vi "REPORT.Max Min P N.vi"(9 "Vasic":i32, 10 "Test":T1={"Config HW"={"VISA Rigol DP832"="Rigol_DP832", "Config Rigol DP832"=[{"Channel"=0, "V Limit"=5.5, "I Limit"=0.5, "V Out"=5.0}, {"Channel"=1, "V Limit"=5.5, "I Limit"=0.8, "V Out"=5.0}, {"Channel"=2, "V Limit"=5.5, "I Limit"=0.2, "V Out"=0.0}], "CTA Test#"="CTA013 A", "FT_Handle"=0, "Espera acceso FT"=10, "VISA Tek MDO3104"="Rigol_DP832", "VISA Key 81160A"="Rigol_DP832"}, "Config Test"=[{"Vasic"=2.8, "Global Reset"=FALSE, "Test Register?"=FALSE, "Test ADC?"=FALSE, "Test ADC"={"Repeats ADC"=100, "Max Desviation"=0.1}, "Limits ADC"={"Low"=[1.9, 1.3, 0.65, 0.0, 1.6, 1.4, 1.4, 0.9, 2.1, 0.85, 1.9], "High"=[2.1, 1.5, 0.85, 0.1, 1.4, 1.2, 1.2, 0.7, 1.9, 0.65, 1.7]}, "Test Max PN Min NP?"=FALSE, "Limits Max PN Min NP"={"Max P Upper"=2.177000045776367, "Min P Upper"=1.474, "Max N Upper"=1.475, "Min N Upper"=0.818, "Max P Lower"=1.888, "Min P Lower "=1.321, "Max N Lower"=1.322, "Min N Lower"=0.73}, "Test Rate Scan?"=FALSE, "Vin Rate Scan"=[], "Limits Rate Scan"={"High"=[0.15, 0.242, 0.331, 0.425, 0.512, 0.6, 0.688, 0.774, 0.847, 0.91], "Low"=[0.021, 0.11, 0.189, 0.27, 0.347, 0.421, 0.487, 0.551, 0.601, 0.635]}, "Test Rate Scan Adders?"=FALSE, "Vin Rate Adders"=[], "Limits Rate Scan adders"={"High"=[], "Low"=[]}, "Test offset analog?"=FALSE, "Lim Offset Analog"={"Max Analog"=0.05, "Min Analog"=-0.05}, "Test offset digital?"=FALSE, "Lim offset Dig"={"Max Dig"=0.05}, "Vasic real f.a."=2.8, "IBIAS"=FALSE, "VALUE IBIAS"=63}, {"Vasic"=2.8, "Global Reset"=FALSE, "Test Register?"=FALSE, "Test ADC?"=FALSE, "Test ADC"={"Repeats ADC"=100, "Max Desviation"=0.1}, "Limits ADC"={"Low"=[1.9, 1.3, 0.65, 0.0, 1.6, 1.4, 1.4, 0.9, 2.1, 0.85, 1.9], "High"=[2.1, 1.5, 0.85, 0.1, 1.4, 1.2, 1.2, 0.7, 1.9, 0.65, 1.7]}, "Test Max PN Min NP?"=FALSE, "Limits Max PN Min NP"={"Max P Upper"=2.177000045776367, "Min P Upper"=1.474, "Max N Upper"=1.475, "Min N Upper"=0.818, "Max P Lower"=1.888, "Min P Lower "=1.321, "Max N Lower"=1.322, "Min N Lower"=0.73}, "Test Rate Scan?"=FALSE, "Vin Rate Scan"=[], "Limits Rate Scan"={"High"=[0.15, 0.242, 0.331, 0.425, 0.512, 0.6, 0.688, 0.774, 0.847, 0.91], "Low"=[0.021, 0.11, 0.189, 0.27, 0.347, 0.421, 0.487, 0.551, 0.601, 0.635]}, "Test Rate Scan Adders?"=FALSE, "Vin Rate Adders"=[], "Limits Rate Scan adders"={"High"=[], "Low"=[]}, "Test offset analog?"=FALSE, "Lim Offset Analog"={"Max Analog"=0.05, "Min Analog"=-0.05}, "Test offset digital?"=FALSE, "Lim offset Dig"={"Max Dig"=0.05}, "Vasic real f.a."=2.8, "IBIAS"=FALSE, "VALUE IBIAS"=63}, {"Vasic"=2.8, "Global Reset"=FALSE, "Test Register?"=FALSE, "Test ADC?"=FALSE, "Test ADC"={"Repeats ADC"=100, "Max Desviation"=0.1}, "Limits ADC"={"Low"=[1.9, 1.3, 0.65, 0.0, 1.6, 1.4, 1.4, 0.9, 2.1, 0.85, 1.9], "High"=[2.1, 1.5, 0.85, 0.1, 1.4, 1.2, 1.2, 0.7, 1.9, 0.65, 1.7]}, "Test Max PN Min NP?"=FALSE, "Limits Max PN Min NP"={"Max P Upper"=2.177000045776367, "Min P Upper"=1.474, "Max N Upper"=1.475, "Min N Upper"=0.818, "Max P Lower"=1.888, "Min P Lower "=1.321, "Max N Lower"=1.322, "Min N Lower"=0.73}, "Test Rate Scan?"=FALSE, "Vin Rate Scan"=[], "Limits Rate Scan"={"High"=[0.15, 0.242, 0.331, 0.425, 0.512, 0.6, 0.688, 0.774, 0.847, 0.91], "Low"=[0.021, 0.11, 0.189, 0.27, 0.347, 0.421, 0.487, 0.551, 0.601, 0.635]}, "Test Rate Scan Adders?"=FALSE, "Vin Rate Adders"=[], "Limits Rate Scan adders"={"High"=[], "Low"=[]}, "Test offset analog?"=FALSE, "Lim Offset Analog"={"Max Analog"=0.05, "Min Analog"=-0.05}, "Test offset digital?"=FALSE, "Lim offset Dig"={"Max Dig"=0.05}, "Vasic real f.a."=2.8, "IBIAS"=FALSE, "VALUE IBIAS"=63}, {"Vasic"=2.8, "Global Reset"=FALSE, "Test Register?"=FALSE, "Test ADC?"=FALSE, "Test ADC"={"Repeats ADC"=100, "Max Desviation"=0.1}, "Limits ADC"={"Low"=[1.9, 1.3, 0.65, 0.0, 1.6, 1.4, 1.4, 0.9, 2.1, 0.85, 1.9], "High"=[2.1, 1.5, 0.85, 0.1, 1.4, 1.2, 1.2, 0.7, 1.9, 0.65, 1.7]}, "Test Max PN Min NP?"=FALSE, "Limits Max PN Min NP"={"Max P Upper"=2.177000045776367, "Min P Upper"=1.474, "Max N Upper"=1.475, "Min N Upper"=0.818, "Max P Lower"=1.888, "Min P Lower "=1.321, "Max N Lower"=1.322, "Min N Lower"=0.73}, "Test Rate Scan?"=FALSE, "Vin Rate Scan"=[], "Limits Rate Scan"={"High"=[0.15, 0.242, 0.331, 0.425, 0.512, 0.6, 0.688, 0.774, 0.847, 0.91], "Low"=[0.021, 0.11, 0.189, 0.27, 0.347, 0.421, 0.487, 0.551, 0.601, 0.635]}, "Test Rate Scan Adders?"=FALSE, "Vin Rate Adders"=[], "Limits Rate Scan adders"={"High"=[], "Low"=[]}, "Test offset analog?"=FALSE, "Lim Offset Analog"={"Max Analog"=0.05, "Min Analog"=-0.05}, "Test offset digital?"=FALSE, "Lim offset Dig"={"Max Dig"=0.05}, "Vasic real f.a."=2.8, "IBIAS"=FALSE, "VALUE IBIAS"=63}], "Result"=[], "Execucion Test"={"Vasic Actual"=0}, "Config VGA"={"Theoretical Voltage"=[], "Real Voltage"=[], "Pulse Width"=57344, "Frecuency Pulse"=1000000.0, "VGA Gain"=[]}, "Test Info"={"Asic"="", "Operator"="", "Place"="", "Time start"=timestamp(0 s since 1904-01-01), "Time stop"=timestamp(0 s since 1904-01-01)}, "Info machine"={"SO"="", "SO Name"="", "SO Ver"="", "SO Build"="", "CPU"="", "APP"="", "APP YEAR"="", "APP ver"="", "APP User"="", "APP Serail"="", "MAC"=[], "PC NAME"=[], "PC IP"=[], "BIOS MANU"="", "BIOS NAME"="", "BIOS SERIAL"="", "BOARD MANU"="", "BOARD NAME"="", "BOARD SERIAL"="", "Driver Version"="", "Library Version"="", "FPGA Ver"=0, "ID CTA board"=0, "LAST BOOT"="", "LABVIEW Ver"=0}, "Partial Report"="", "CONFIG GEN"=[]} {"CONFIG GEN"."Vasic Theorical" min=1.0 max=1000000.0 step=1.0 format="%#_6pV"; "CONFIG GEN"."Frequency" min=0.001 max=333000000.0 step=1000.0 format="%#_6pHz"; "CONFIG GEN"."Leading Edge Time" min=1e-09 max=1.0 step=1e-10 format="%#_6ps"; "CONFIG GEN"."Trailing Edge Time" min=1e-09 max=1.0 step=1e-10 format="%#_6ps"; "CONFIG GEN"."Delay" min=0.0 max=1.0 step=1e-12 format="%#_6ps"; "CONFIG GEN"."Trigger Level Sync" items=["ECL", "TTL"]; "CONFIG GEN"."Trigger Sync Out" items=["AB"=3, "B"=2, "A"=1, "None"=0]; "CONFIG GEN"."Load" min=1.0 max=1000000.0 step=1.0 format="%#_6p"; "CONFIG GEN"."DC Offset" min=-10.0 max=10.0 step=0.1 format="%#_6pV"; "CONFIG GEN"."Amplitude" min=0.05 max=5.0 step=0.001 format="%#_6pV"; "CONFIG GEN"."Width Time" min=1.5e-09 max=1.0 step=1e-10 format="%#_6ps"; "CONFIG GEN"."Channel" items=["Channel1"=1, "Channel2"=2]; "Config VGA"."Theoretical Voltage" format="%1.4f"; "Config VGA"."VGA Gain" format="%02x"; "Config VGA"."Frecuency Pulse" format="%0_2p"; "Config VGA"."Pulse Width" format="%04x"; "Config VGA"."Real Voltage" format="%1.5f"; "Config Test"."VALUE IBIAS" max=63 step=1; "Config Test"."Vasic real f.a." min=2.8 max=3.8 step=0.01 format="%.2g"; "Config Test"."Limits Rate Scan adders"."Low" format="%1.3f"; "Config Test"."Limits Rate Scan adders"."High" format="%1.3f"; "Config Test"."Limits ADC"."High" format="%1.4f"; "Config Test"."Limits ADC"."Low" format="%1.3f"; "Config Test"."Lim offset Dig"."Max Dig" format="%.3g"; "Config Test"."Lim Offset Analog"."Min Analog" format="%.3g"; "Config Test"."Lim Offset Analog"."Max Analog" format="%.3g"; "Config Test"."Limits Rate Scan"."Low" format="%1.4f"; "Config Test"."Limits Rate Scan"."High" format="%1.3f"; "Config Test"."Limits Max PN Min NP"."Min P Upper" format="%.3g"; "Config Test"."Limits Max PN Min NP"."Min P Lower" format="%.3g"; "Config Test"."Limits Max PN Min NP"."Max N Lower" format="%.3g"; "Config Test"."Limits Max PN Min NP"."Max N Upper" format="%.3g"; "Config Test"."Limits Max PN Min NP"."Min N Lower" format="%.3g"; "Config Test"."Limits Max PN Min NP"."Min N Upper" format="%.3g"; "Config Test"."Limits Max PN Min NP"."Max P Upper" format="%.3g"; "Config Test"."Limits Max PN Min NP"."Max P Lower" format="%.3g"; "Config Test"."Vasic" min=2.8 max=3.8 step=0.01 format="%.2g"; "Config HW"."Config Rigol DP832"."Channel" items=["+30V Channel 1", "+30V Channel 2", "+5V Channel 3"]; "Config HW"."Config Rigol DP832"."V Limit" format="%.1g"; "Config HW"."Config Rigol DP832"."I Limit" format="%.1g"; "Config HW"."Config Rigol DP832"."V Out" format="%.1g"; "Result"."Test Registros"."Read W/R" format="%04x"; "Result"."Test Registros"."Pattern W/R" format="%04x"; "Result"."Test Registros"."Read Default" format="%04x"; "Result"."Test Registros"."Pattern Default" format="%04x"}, 11 "Text in":string) -> (3 "Text Out":string)   [LabVIEW 2019]
uses:
  Test.ctl
  TEST.TEST CONFIG HW.ctl
  Rigol DP832/DP832_Control Channels.ctl
  TEST.TEST CONFIG TEST MATRIZ.ctl
  TEST.TEST CONFIG TEST.ctl
  TEST.TEST RESULT.ctl
  test_result fvasic.ctl
  TEST.TEST EXECUTION TEST.ctl
  TEST.TEST CONFIG VGA.ctl
  TEST.TEST TEST INFO.ctl
  TEST.TEST INFO PC.ctl
  GenPulse_configurar.ctl
panel:
  # "Modo 2\nModo 3\nModo 4\nModo 2\nModo 3\nModo 4"
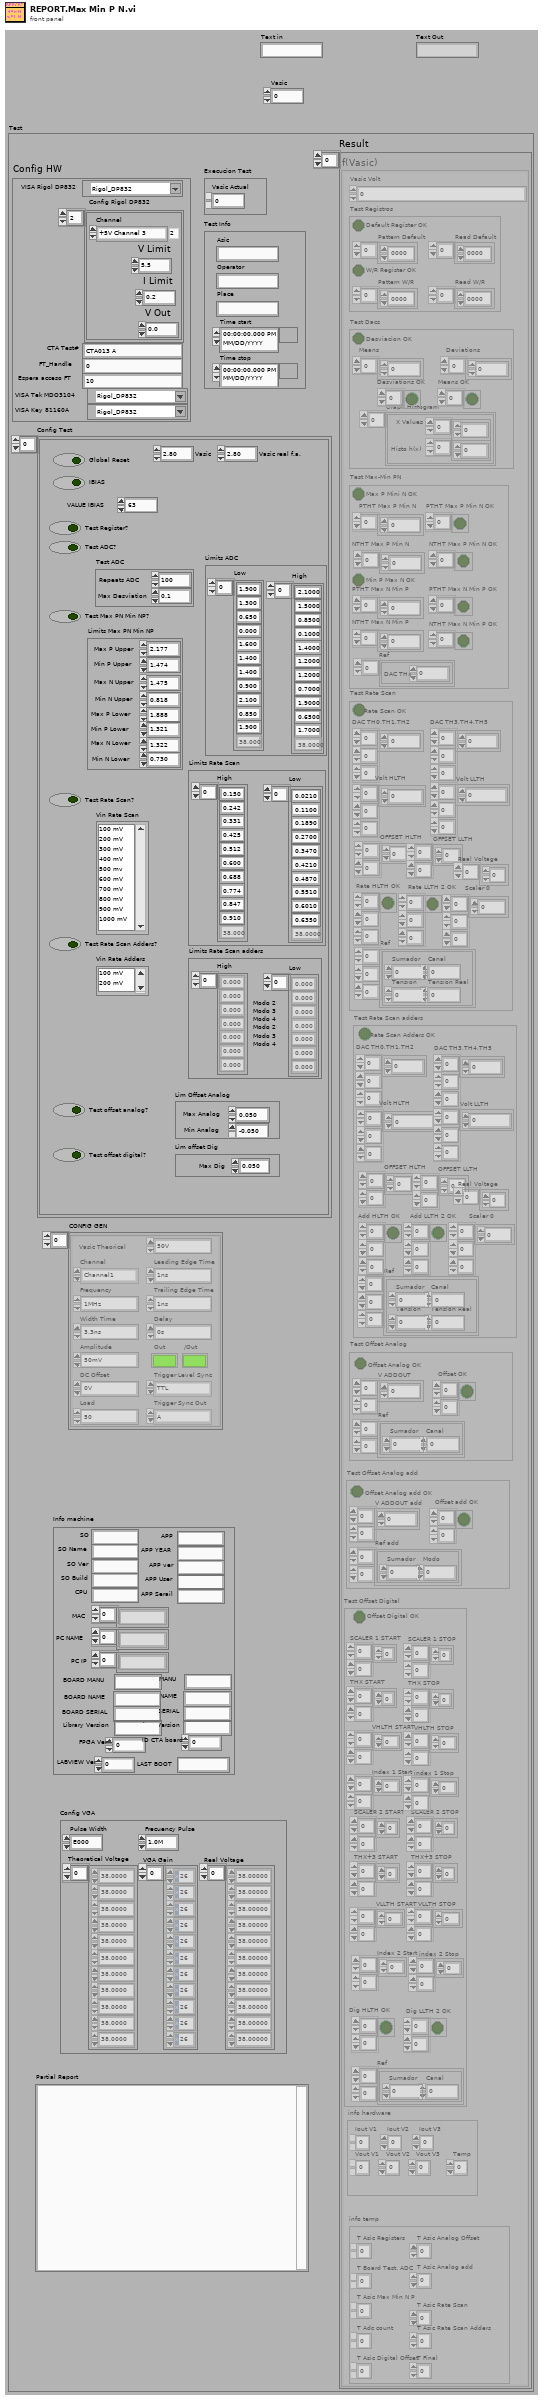
[diagram p1: front panel]
types:
  T1 = typedef "Test.ctl" = cluster{"Config HW":T2, "Config Test":T4, "Result":T6, "Execucion Test":T8, "Config VGA":T9, "Test Info":T10, "Info machine":T11, "Partial Report":string, "CONFIG GEN":T12[]}
  T2 = typedef "TEST.TEST CONFIG HW.ctl" = cluster{"VISA Rigol DP832":refnum<visa-resource-name>, "Config Rigol DP832":cluster{"Channel":T3, "V Limit":dbl, "I Limit":dbl, "V Out":dbl}[], "CTA Test#":string, "FT_Handle":u32, "Espera acceso FT":u32, "VISA Tek MDO3104":refnum<visa-resource-name>, "VISA Key 81160A":refnum<visa-resource-name>}
  T3 = typedef "DP832_Control Channels.ctl" = i32
  T4 = typedef "TEST.TEST CONFIG TEST MATRIZ.ctl" = T5[]
  T5 = typedef "TEST.TEST CONFIG TEST.ctl" = cluster{"Vasic":dbl, "Global Reset":bool, "Test Register?":bool, "Test ADC?":bool, "Test ADC":cluster{"Repeats ADC":i32, "Max Desviation":dbl}, "Limits ADC":cluster{"Low":dbl[], "High":dbl[]}, "Test Max PN Min NP?":bool, "Limits Max PN Min NP":cluster{"Max P Upper":dbl, "Min P Upper":dbl, "Max N Upper":dbl, "Min N Upper":dbl, "Max P Lower":dbl, "Min P Lower ":dbl, "Max N Lower":dbl, "Min N Lower":dbl}, "Test Rate Scan?":bool, "Vin Rate Scan":i32[], "Limits Rate Scan":cluster{"High":dbl[], "Low":dbl[]}, "Test Rate Scan Adders?":bool, "Vin Rate Adders":i32[], "Limits Rate Scan adders":cluster{"High":dbl[], "Low":dbl[]}, "Test offset analog?":bool, "Lim Offset Analog":cluster{"Max Analog":dbl, "Min Analog":dbl}, "Test offset digital?":bool, "Lim offset Dig":cluster{"Max Dig":dbl}, "Vasic real f.a.":dbl, "IBIAS":bool, "VALUE IBIAS":u8}
  T6 = typedef "TEST.TEST RESULT.ctl" = T7[]
  T7 = typedef "test_result fvasic.ctl" = cluster{"Vasic Volt":i32, "Test Registros":cluster{"Default Register OK":bool, "Pattern Default":u16[], "Read Default":u16[], "W/R Register OK":bool, "Pattern W/R":u16[], "Read W/R":u16[]}, "Test Dacs":cluster{"Desviacion OK":bool, "Means":dbl[], "Deviations":dbl[], "Desviations OK":bool[], "Means OK":bool[], "Graph Histogram":cluster{"X Values":dbl[], "Histo h(x)":i32[]}[]}, "Test Max-Min PN":cluster{"Max P Mini N OK":bool, "PTHT Max P Min N":dbl[], "PTHT Max P Min N OK":bool[], "NTHT Max P Min N":dbl[], "NTHT Max P Min N OK":bool[], "Min P Max N OK":bool, "PTHT Max N Min P":dbl[], "PTHT Max N Min P OK":bool[], "NTHT Max N Min P":dbl[], "NTHT Max N Min P OK":bool[], "Ref":cluster{"DAC THx":u8}[]}, "Test Rate Scan":cluster{"Rate Scan OK":bool, "DAC TH0,TH1,TH2":u16[][][], "Volt HLTH":dbl[][][], "Rate HLTH OK":bool[][][], "DAC TH3,TH4,TH5":u16[][][], "Volt LLTH":dbl[][][], "Rate LLTH 2 OK":bool[][][], "Scaler 0":u16[][][], "Ref":cluster{"Sumador":u8, "Canal":u8, "Tension":u8, "Tension Real":dbl}[][][], "OFFSET HLTH":dbl[][], "OFFSET LLTH":dbl[][], "Real Voltage":dbl[]}, "Test Rate Scan adders":cluster{"Rate Scan Adders OK":bool, "DAC TH0,TH1,TH2":u16[][][], "Volt HLTH":dbl[][][], "Add HLTH OK":bool[][][], "DAC TH3,TH4,TH5":u16[][][], "Volt LLTH":dbl[][][], "Add LLTH 2 OK":bool[][][], "Scaler 0":u16[][][], "Ref":cluster{"Sumador":u8, "Canal":u8, "Tension":u8, "Tension Real":dbl}[][][], "OFFSET HLTH":dbl[][], "OFFSET LLTH":dbl[][], "Real Voltage":dbl[]}, "Test Offset Analog":cluster{"Offset Analog OK":bool, "V ADDOUT":dbl[][], "Offset OK":bool[][], "Ref":cluster{"Sumador":u8, "Canal":u8}[][]}, "Test Offset Digital":cluster{"Offset Digital OK":bool, "SCALER 1 START":u16[][], "SCALER 1 STOP":u16[][], "THX START":u16[][], "THX STOP":u16[][], "VHLTH START":dbl[][], "VHLTH STOP":dbl[][], "Index 1 Start":i32[][], "index 1 Stop":i32[][], "SCALER 2 START":u16[][], "SCALER 2 STOP":u16[][], "THX+3 START":u16[][], "THX+3 STOP":u16[][], "VLLTH START":dbl[][], "VLLTH STOP":dbl[][], "Index 2 Start":i32[][], "index 2 Stop":i32[][], "Dig HLTH OK":bool[][], "Dig LLTH 2 OK":bool[][], "Ref":cluster{"Sumador":u8, "Canal":u8}[][]}, "info hardware":cluster{"Iout V1":dbl, "Iout V2":dbl, "Iout V3":dbl, "Vout V1":dbl, "Vout V2":dbl, "Vout V3":dbl, "Temp":dbl}, "Test Offset Analog add":cluster{"Offset Analog add OK":bool, "V ADDOUT add":dbl[][], "Offset add OK":bool[][], "Ref add":cluster{"Sumador":u8, "Modo":u8}[][]}, "info temp":cluster{"T Asic Registers":dbl, "T Board Test. ADC":dbl, "T Asic Max Min N P":dbl, "T Adc count":dbl, "T Asic Digital Offset":dbl, "T Asic Analog Offset":dbl, "T Asic Analog add":dbl, "T Asic Rate Scan":dbl, "T Asic Rate Scan Adders":dbl, "T Final":dbl}}
  T8 = typedef "TEST.TEST EXECUTION TEST.ctl" = cluster{"Vasic Actual":i32}
  T9 = typedef "TEST.TEST CONFIG VGA.ctl" = cluster{"Theoretical Voltage":dbl[], "Real Voltage":dbl[], "Pulse Width":u16, "Frecuency Pulse":dbl, "VGA Gain":u8[]}
  T10 = typedef "TEST.TEST TEST INFO.ctl" = cluster{"Asic":string, "Operator":string, "Place":string, "Time start":timestamp, "Time stop":timestamp}
  T11 = typedef "TEST.TEST INFO PC.ctl" = cluster{"SO":string, "SO Name":string, "SO Ver":string, "SO Build":string, "CPU":string, "APP":string, "APP YEAR":string, "APP ver":string, "APP User":string, "APP Serail":string, "MAC":string[], "PC NAME":string[], "PC IP":string[], "BIOS MANU":string, "BIOS NAME":string, "BIOS SERIAL":string, "BOARD MANU":string, "BOARD NAME":string, "BOARD SERIAL":string, "Driver Version":string, "Library Version":string, "FPGA Ver":u8, "ID CTA board":u64, "LAST BOOT":string, "LABVIEW Ver":u32}
  T12 = typedef "GenPulse_configurar.ctl" = cluster{"Channel":u16, "Frequency":dbl, "Width Time":dbl, "Amplitude":dbl, "DC Offset":dbl, "Load":dbl, "Leading Edge Time":dbl, "Trailing Edge Time":dbl, "Delay":dbl, "Out":bool, "/Out":bool, "Trigger Level Sync":u16, "Trigger Sync Out":u16, "Vasic Theorical":dbl}
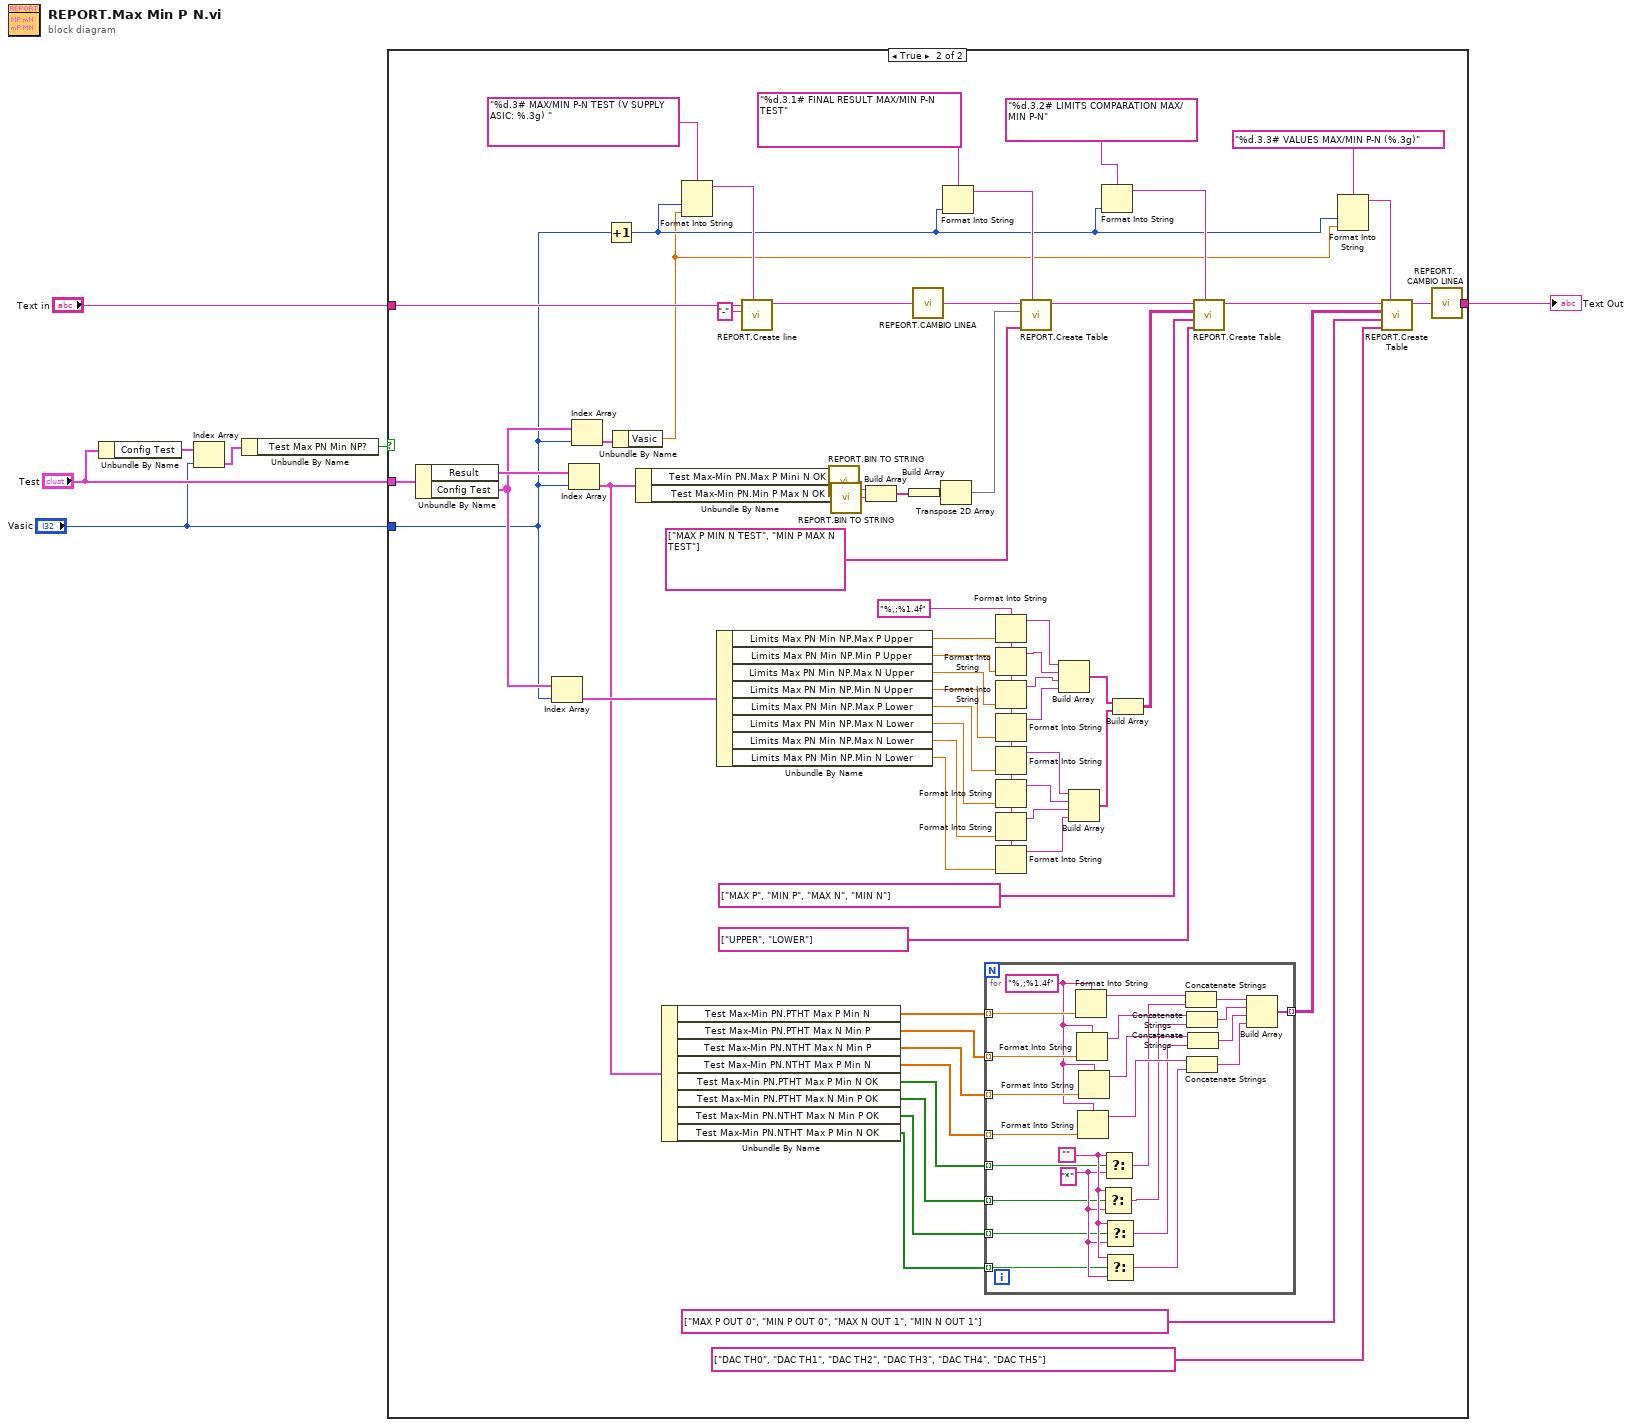
[diagram p0: block diagram]
diagram:
  n1 = Unbundle By Name("Test") -> ("Config Test"=w5:T4)
  n2 = Index Array(array=w5, index="Vasic") -> (element=w4:T5)
  n3 = Unbundle By Name(w4) -> ("Test Max PN Min NP?"=w1:bool)
  n4 = case shown="True" w1 {
    tunnel: "Text in" -> [w8 w68]
    tunnel: [w8 w24] -> w6
    tunnel: "Test" -> [_ w12]
    tunnel: "Vasic" -> [_ w11]
    frame False {
    }
    frame True {
      w43 = "%,;%1.4f" ("format string")
      n5 = Unbundle By Name(w12) -> ("Result"=w67:T6, "Config Test"=w19:T4)
      n6 = Index Array(array=w19, index=w11) -> (element=w64:T5)
      n7 = Index Array(array=w67, index=w11) -> (element=w39:T7)
      n8 = Index Array(array=w19, index=w11) -> (element=w18:T5)
      n9 = Increment(x=w11) -> (x+1=w13:i32)
      n10 = Unbundle By Name(w18) -> ("Vasic"=w10:dbl)
      n11 = Unbundle By Name(w39) -> ("Test Max-Min PN.Max P Mini N OK"=w72:bool, "Test Max-Min PN.Min P Max N OK"=w73:bool)
      n12 = Unbundle By Name(w39) -> ("Test Max-Min PN.PTHT Max P Min N"=w38:dbl[], "Test Max-Min PN.PTHT Max N Min P"=w37:dbl[], "Test Max-Min PN.NTHT Max N Min P"=w36:dbl[], "Test Max-Min PN.NTHT Max P Min N"=w35:dbl[], "Test Max-Min PN.PTHT Max P Min N OK"=w31:bool[], "Test Max-Min PN.PTHT Max N Min P OK"=w30:bool[], "Test Max-Min PN.NTHT Max N Min P OK"=w29:bool[], "Test Max-Min PN.NTHT Max P Min N OK"=w28:bool[])
      n13 = Format Into String(format string="%d.3# MAX/MIN P-N TEST (V SUPPLY ASIC: %.3g) " ("Secction"), w13, w10) -> (resulting string=w17:string)  [unwired: 2 in, 1 out]
      n14 = Unbundle By Name(w64) -> ("Limits Max PN Min NP.Max P Upper"=w63:dbl, "Limits Max PN Min NP.Min P Upper"=w62:dbl, "Limits Max PN Min NP.Max N Upper"=w61:dbl, "Limits Max PN Min NP.Min N Upper"=w60:dbl, "Limits Max PN Min NP.Max P Lower"=w59:dbl, "Limits Max PN Min NP.Max N Lower"=w58:dbl, "Limits Max PN Min NP.Max N Lower"=w57:dbl, "Limits Max PN Min NP.Min N Lower"=w56:dbl)
      n15 = call "REPORT.Create line.vi"("Secction"=w17, "Char"="-", "Text In"=w68) -> ("Text Out"=w55:string)  [unwired: 8 in]
      n16 = call "REPORT.BIN TO STRING.vi"("Resultado test"=w72) -> ("OK, Fault"=w71:string)  [unwired: 14 in]
      n17 = call "REPORT.BIN TO STRING.vi"("Resultado test"=w73) -> ("OK, Fault"=w70:string)  [unwired: 14 in]
      n18 = Build Array(w71, w70) -> (w69:string[])
      n19 = Build Array(w69) -> (w74:string[][])
      n20 = call "REPEORT.CAMBIO LINEA.vi"("Text Out"=w55) -> ("String"=w54:string)  [unwired: 8 in]
      n21 = Transpose 2D Array(2D array=w74) -> (transposed array=w66:string[][])
      n22 = Format Into String(format string="%d.3.1# FINAL RESULT MAX/MIN P-N TEST" ("Secction"), w13) -> (resulting string=w16:string)  [unwired: 2 in, 1 out]
      n23 = for {
        tunnel: w38 -> [w98] mode=indexing
        tunnel: w37 -> [w97] mode=indexing
        tunnel: w36 -> [w96] mode=indexing
        tunnel: w35 -> [w95] mode=indexing
        tunnel: [w93] -> w34 mode=indexing
        tunnel: w31 -> [w90] mode=indexing
        tunnel: w30 -> [w89] mode=indexing
        tunnel: w29 -> [w88] mode=indexing
        tunnel: w28 -> [w87] mode=indexing
        w91 = "*"
        w92 = ""
        w94 = "%,;%1.4f" ("format string")
        n24 = Format Into String(format string=w94, w98) -> (resulting string=w86:string)  [unwired: 2 in, 1 out]
        n25 = Format Into String(format string=w94, w97) -> (resulting string=w85:string)  [unwired: 2 in, 1 out]
        n26 = Format Into String(format string=w94, w95) -> (resulting string=w83:string)  [unwired: 2 in, 1 out]
        n27 = Format Into String(format string=w94, w96) -> (resulting string=w84:string)  [unwired: 2 in, 1 out]
        n28 = Select(t=w92, s=w89, f=w91) -> (s? t:f=w77:string)
        n29 = Select(t=w92, s=w90, f=w91) -> (s? t:f=w82:string)
        n30 = Select(t=w92, s=w88, f=w91) -> (s? t:f=w76:string)
        n31 = Select(t=w92, s=w87, f=w91) -> (s? t:f=w75:string)
        n32 = Concatenate Strings(w86, w82) -> (w81:string)
        n33 = Concatenate Strings(w85, w77) -> (w80:string)
        n34 = Concatenate Strings(w83, w75) -> (w78:string)
        n35 = Concatenate Strings(w84, w76) -> (w79:string)
        n36 = Build Array(w81, w80, w79, w78) -> (w93:string[])
      }
      n37 = Format Into String(format string=w43, w63) -> (resulting string=w51:string)  [unwired: 2 in, 1 out]
      n38 = Format Into String(format string=w43, w62) -> (resulting string=w50:string)  [unwired: 2 in, 1 out]
      n39 = Format Into String(format string=w43, w61) -> (resulting string=w49:string)  [unwired: 2 in, 1 out]
      n40 = Format Into String(format string=w43, w60) -> (resulting string=w48:string)  [unwired: 2 in, 1 out]
      n41 = Format Into String(format string=w43, w59) -> (resulting string=w47:string)  [unwired: 2 in, 1 out]
      n42 = Format Into String(format string=w43, w58) -> (resulting string=w46:string)  [unwired: 2 in, 1 out]
      n43 = Format Into String(format string=w43, w57) -> (resulting string=w45:string)  [unwired: 2 in, 1 out]
      n44 = Format Into String(format string=w43, w56) -> (resulting string=w44:string)  [unwired: 2 in, 1 out]
      n45 = call "REPORT.Create Table.vi"("Secction"=w16, "Row Headers"=string[] ["MAX P MIN N TEST", "MIN P MAX N TEST"], "Text 2d"=w66, "Text In"=w54) -> ("Text Out"=w27:string)  [unwired: 4 in, 1 out]
      n46 = Build Array(w51, w50, w49, w48) -> (w41:string[])
      n47 = Build Array(w47, w46, w45, w44) -> (w42:string[])
      n48 = Format Into String(format string="%d.3.2# LIMITS COMPARATION MAX/MIN P-N" ("Secction"), w13) -> (resulting string=w15:string)  [unwired: 2 in, 1 out]
      n49 = Build Array(w41, w42) -> (w40:string[][])
      n50 = call "REPORT.Create Table.vi"("Secction"=w15, "Row Headers"=string[] ["UPPER", "LOWER"] ("Column Headers"), "Column Headers"=string[] ["MAX P", "MIN P", "MAX N", "MIN N"], "Text 2d"=w40, "Text In"=w27) -> ("Text Out"=w26:string)  [unwired: 3 in, 1 out]
      n51 = Format Into String(format string="%d.3.3# VALUES MAX/MIN P-N (%.3g)" ("Secction"), w13, w10) -> (resulting string=w14:string)  [unwired: 2 in, 1 out]
      n52 = call "REPORT.Create Table.vi"("Secction"=w14, "Row Headers"=string[] ["DAC TH0", "DAC TH1", "DAC TH2", "DAC TH3", "DAC TH4", "DAC TH5"] ("Column Headers"), "Column Headers"=string[] ["MAX P OUT 0", "MIN P OUT 0", "MAX N OUT 1", "MIN N OUT 1"], "Text 2d"=w34, "Text In"=w26) -> ("Text Out"=w25:string)  [unwired: 3 in, 1 out]
      n53 = call "REPEORT.CAMBIO LINEA.vi"("Text Out"=w25) -> ("String"=w24:string)  [unwired: 8 in]
    }
  }
  "Text Out" <- w6
